vi "Navigation Variables.vi"() -> ()   [LabVIEW 2016, in "Shared resources RT.lvlib"]
uses:
  Shared resources RT.lvlib
panel:
  out "FIltered Yaw":dbl
  out "UsePath":bool
  out "RemoteSetpoint":dbl
  out "SetNav":bool
  out "Lean Angle":dbl
  out "Setpoint":dbl
  out "Increment Lean":i8
  out "Steering Angle [deg]":dbl
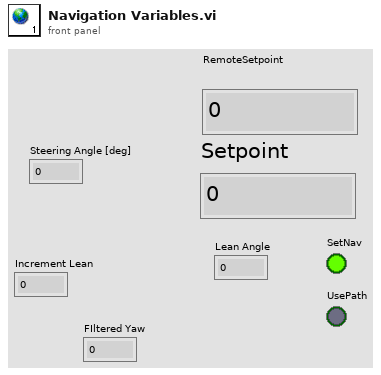
[diagram p1: front panel]
diagram:
